vi "Example.vi"() -> ()   [LabVIEW 2015, in "Vaisala.lvclass"]
uses:
  Vaisala.lvclass
  Reusable/Session APIs/File Access/Config Data/Config Data.lvclass
  Instruments/Nicholas/Session/FPGA Serial Session.lvclass
  Instruments/Nicholas/Session/Raw FPGA/FPGA Session.lvclass
  Reusable/Session Log/System Log.lvclass
  Reusable/Session APIs/File Access/Config Data/Config Session.ctl
  Reusable/Session Log/System Log.lvclass/System Log.ctl
  Reusable/Session APIs/File Access/Config Data/Config Data.lvclass/Config Data.ctl
  Instruments/Nicholas/Session/Raw FPGA/FPGA Session.lvclass/FPGA Session.ctl
  Instruments/Nicholas/Session/FPGA Serial Session.lvclass/FPGA Serial Session.ctl
  Reusable/Session APIs/Text Communication/Text Device Session.lvclass/Text Device Session.ctl
  Configurable Device/Configurable Device.lvclass/Configurable Device.ctl
  Vaisala.lvclass/Vaisala.ctl
  Reusable/Session Log/Accessors/Write Main Path.vi
  Instruments/Nicholas/Session/Raw FPGA/Read FPGA Ref.vi
  Reusable/Session APIs/File Access/Config Data/Accessors/Write Cfg Path.vi
  Instruments/Nicholas/Session/Write fpgaSession.vi
  Reusable/Session APIs/Text Communication/Write hSysLog.vi
  Configurable Device/Write Handle.vi
  Accessors/Write hSession.vi
  Accessors/Write ID.vi
  <vilib>/Utility/error.llb/Error Cluster From Error Code.vi
  <vilib>/RVI Host/nirviSupport.llb/nirviErrorClusterFromErrorCode.vi
  <vilib>/rvi/errors/niLvFpgaAdjustHostInterfaceError.vi
  Reusable/Data/Array Data/Single 1-D/Read Data.vi
  Instruments/Nicholas/FPGA Ref.ctl
  <vilib>/rvi/interface/nirviMethod/nirviMethod.xnode
  Instruments/Nicholas/FPGA Bitfiles/NickIO.lvbitx
  <vilib>/rvi/interface/nirviReadWriteControl/nirviReadWriteControl.xnode
  <userlib>/_Session Fwk/Session - Root.lvclass
  Reusable/Data/Array Data/Single 1-D/Single_Array.lvclass
  <vilib>/rvi/interface/nirviMethod/StockFPGA_InlinedMethodWaitForSingleIRQ.vi
  <vilib>/FPGAPlugInAG/cRIO-9081/niLvFpga_WaitOnIrq_cRIO-9081.vi
  <vilib>/FPGAPlugInAG/cRIO-9081/niLvFpga_AcknowledgeIrq_cRIO-9081.vi
  NiFpgaLv.dll
panel:
  out "Data":sgl[](array[numeric])
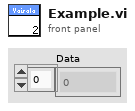
[diagram p1: front panel]
types:
  T1 = typedef "Config Data.lvclass/Config Session.ctl" = refnum<data-value>
  T2 = typedef "Session - Root.lvclass/Session Handle.ctl" = refnum<data-value>
  T3 = typedef "FPGA Ref.ctl" = refnum<k20>
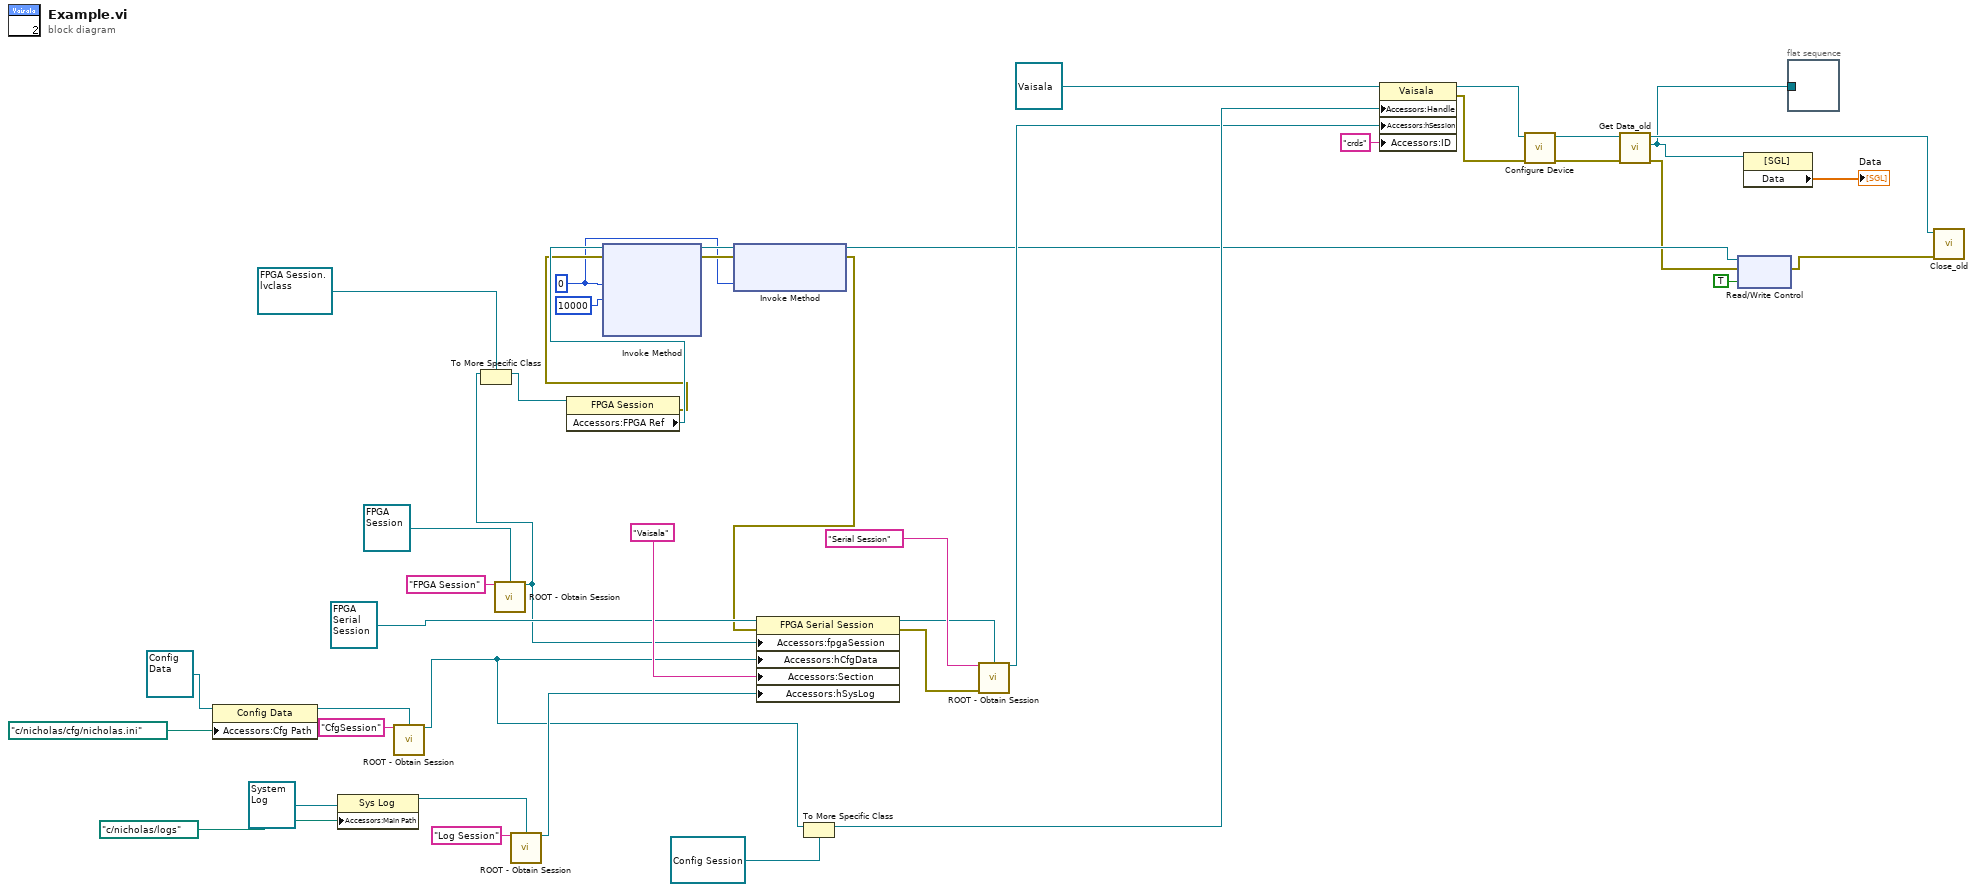
[diagram p0: block diagram]
diagram:
  w18 = 0 ("IRQ Number(s)")
  n1 = property class="Config Data"(reference=refnum<class "Config Data.lvclass"> refnum ("Config Data"), "Accessors:Cfg Path"=path "c:/nicholas/cfg/nicholas.ini" ("Cfg Path")) -> (reference out=w40:refnum<class "Config Data.lvclass">)  [unwired: 1 in, 1 out]
  n2 = property class="Sys Log"(reference=refnum<class "System Log.lvclass"> refnum ("Sys Log"), "Accessors:Main Path"=path "c:/nicholas/logs" ("Main Path")) -> (reference out=w29:refnum<class "System Log.lvclass">)  [unwired: 1 in, 1 out]
  n3 = call <userlib>:"ROOT - Obtain Session.vi"("Session Name ()"="CfgSession", "OBJ - Session"=w40) -> ("Session Handle"=w16:T2)  [unwired: 11 in, 2 out]
  n4 = call <userlib>:"ROOT - Obtain Session.vi"("Session Name ()"="FPGA Session", "OBJ - Session"=refnum<class "FPGA Session.lvclass"> refnum ("FPGA Session.lvclass")) -> ("Session Handle"=w25:T2)  [unwired: 11 in, 2 out]
  n5 = To More Specific Class(target class=refnum<data-value> refnum ("Session Handle"), reference=w25) -> (specific class reference=w23:refnum<data-value>)  [unwired: 1 in, 1 out]
  n6 = call <userlib>:"ROOT - Obtain Session.vi"("Session Name ()"="Log Session", "OBJ - Session"=w29) -> ("Session Handle"=w32:T2)  [unwired: 11 in, 2 out]
  n7 = property class="FPGA Session"(reference=w23) -> (error out=w19:errorcluster, "Accessors:FPGA Ref"=w20:T3)  [unwired: 1 in, 1 out]
  n8 = xnode "Invoke Method"("FPGA VI Reference In"=w20, "error in"=w19, "IRQ Number(s)"=w18, "Timeout (ms)"=10000) -> ("FPGA VI Reference Out"=w22:T3, "error out"=w21:errorcluster)  [unwired: 2 out]
  n9 = xnode "Invoke Method"("FPGA VI Reference In"=w22, "error in"=w21, "IRQ Number(s)"=w18) -> ("FPGA VI Reference Out"=w6:T3, "error out"=w17:errorcluster)
  n10 = property class="FPGA Serial Session"(reference=refnum<class "FPGA Serial Session.lvclass"> refnum ("FPGA Serial Session.lvclass"), error in=w17, "Accessors:fpgaSession"=w25, "Accessors:hCfgData"=w16, "Accessors:Section"="Vaisala" ("Section"), "Accessors:hSysLog"=w32) -> (reference out=w35:refnum<class "FPGA Serial Session.lvclass">, error out=w27:errorcluster)
  n11 = To More Specific Class(target class=T1 refnum ("Handle"), reference=w16) -> (specific class reference=w14:T1)  [unwired: 1 in, 1 out]
  n12 = call <userlib>:"ROOT - Obtain Session.vi"("Session Name ()"="Serial Session", "OBJ - Session"=w35, "error in (no error)"=w27) -> ("Session Handle"=w13:T2)  [unwired: 10 in, 2 out]
  n13 = property class="Vaisala"(reference=refnum<class "Vaisala.lvclass"> refnum ("Vaisala"), "Accessors:Handle"=w14, "Accessors:hSession"=w13, "Accessors:ID"="crds" ("ID")) -> (reference out=w11:refnum<class "Vaisala.lvclass">, error out=w10:errorcluster)  [unwired: 1 in]
  n14 = call-dynamic "Configure Device.vi"("error in"=w10, "Vaisala Probe in"=w11) -> ("error out"=w8:errorcluster, "Vaisala Probe out"=w9:refnum<class "Vaisala.lvclass">)  [unwired: 8 in]
  n15 = call "Get Data_old.vi"("error in"=w8, "Vaisala Probe in"=w9) -> ("error out"=w5:errorcluster, "Data Out"=w1:refnum<class "Single_Array.lvclass">, "Vaisala Probe out"=w3:refnum<class "Vaisala.lvclass">)  [unwired: 7 in]
  n16 = xnode "Read/Write Control"("FPGA VI Reference In"=w6, "error in"=w5, "Stop"=TRUE) -> ("error out"=w4:errorcluster)  [unwired: 1 out]
  n17 = property class="[SGL]"(reference=w1) -> ("Data"=→"Data":sgl[])  [unwired: 1 in, 2 out]
  n18 = flat-sequence {
    tunnel: w1 -> [_]
    frame #0 {
    }
  }
  n19 = call "Close_old.vi"("error in (no error)"=w4, "Vaisala in"=w3) -> ()  [unwired: 8 in, 2 out]
